vi "Config.Simulate.Check.vi"(11 "Config Folder":path=path "C:/DDCS/Config") -> (3 "Simulate":bool)   [LabVIEW 2024, in "EQMF.lvlib" / "Config Utils.lvlib"]
doc: "This VI reads the simulate flag (Boolean) from the station config INI file (Local Station.ini).\nThe Simulate flag is stored in section \"Simulate\" item \"Enable\".\n\nINPUTS:\n<B>Config folder</B> - This is the folder where config files are stored.\n\nOUTPUTS:\n<B>Simulate</B> - TRUE means simulate mode is ON.\n\nERRORS: \nNo errors will be reported. If the config file cannot be read, the Simulate flag will be set to FALSE."
uses:
  Config Utils.lvlib
  <vilib>/Utility/config.llb/Read Key (Boolean).vi
  <vilib>/Utility/config.llb/Write Key (Boolean).vi
  <vilib>/Utility/config.llb/NI_LVConfig.lvlib
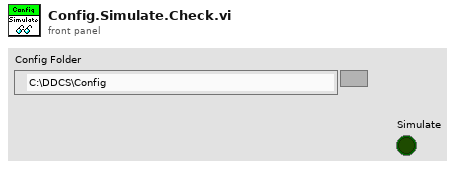
[diagram p1: front panel]
types:
  T1 = typedef "NI_LVConfig.lvlib/Config Data RefNum.ctl" = refnum<k1>
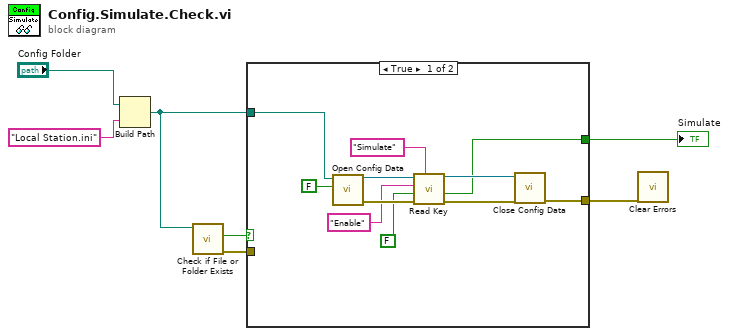
[diagram p0: block diagram]
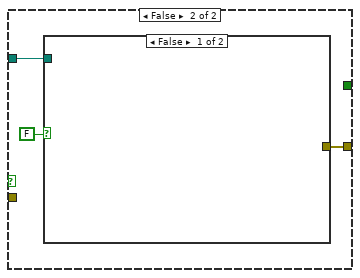
[diagram p2: hidden frame]
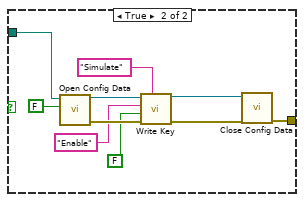
[diagram p3: hidden frame]
diagram:
  n1 = Build Path(base path="Config Folder", name or relative path="Local Station.ini") -> (appended path=w4:path)
  n2 = call <vilib>:"Check if File or Folder Exists.vi"("path"=w4) -> ("error out"=w2:errorcluster, "file or folder exists?"=w3:bool)  [unwired: 8 in, 1 out]
  n3 = case shown="True" w3 {
    tunnel: [w10 _] -> w6
    tunnel: [w9 w21] -> w5
    tunnel: w4 -> [w8 w20]
    tunnel: w2 -> [_ _]
    frame True {
      n4 = call <vilib>:"Open Config Data.vi"("create file if necessary (T)"=FALSE, "configuration file path"=w8) -> ("error out"=w16:errorcluster, "refnum"=w17:T1)  [unwired: 7 in, 1 out]
      n5 = call-poly <vilib>:"Read Key.vi"("section"="Simulate", "error in (no error)"=w16, "default value"=FALSE, "key"="Enable", "refnum"=w17) -> ("error out"=w12:errorcluster, "value"=w10:bool, "refnum out"=w13:T1)  [unwired: 3 in, 1 out]
      n6 = call <vilib>:"Close Config Data.vi"("error in (no error)"=w12, "refnum"=w13) -> ("error out"=w9:errorcluster)  [unwired: 8 in, 1 out]
    }
    frame False {
      n7 = case shown="False" FALSE {
        tunnel: [_ w23] -> w21
        tunnel: w20 -> [_ w22]
        frame False {
        }
        frame True {
          n8 = call <vilib>:"Open Config Data.vi"("create file if necessary (T)"=FALSE, "configuration file path"=w22) -> ("error out"=w29:errorcluster, "refnum"=w30:T1)  [unwired: 7 in, 1 out]
          n9 = call-poly <vilib>:"Write Key.vi"("section"="Simulate", "error in (no error)"=w29, "value"=FALSE ("default value"), "key"="Enable", "refnum"=w30) -> ("error out"=w25:errorcluster, "refnum out"=w26:T1)  [unwired: 4 in, 1 out]
          n10 = call <vilib>:"Close Config Data.vi"("error in (no error)"=w25, "refnum"=w26) -> ("error out"=w23:errorcluster)  [unwired: 8 in, 1 out]
        }
      }
    }
  }
  "Simulate" <- w6
  n11 = call <vilib>:"Clear Errors.vi"("error in (no error)"=w5) -> ()  [unwired: 5 in, 2 out]
